vi "Modes of operation.vi"(8 "error in (no error)":errorcluster, 9 "W/R":enum16{"Write", "Read"}(ring), 10 "Ring":i8(ring) items=["No mode change/no mode assigned"=0, "Profile position mode"=1, "Velocity mode"=2, "Profile velocity mode"=3, "Torque profile mode"=4, "Homing mode"=6, "Interpolated position mode"=7, "Cyclic synchronous position mode"=8, "Cyclic synchronous velocity mode"=9, "Cyclic synchronous torque mode"=10], 11 "Motor Base in":refnum<class "Motor Base.lvclass">) -> (0 "error out":errorcluster, 2 "Ring":i8(ring) items=["No mode change/no mode assigned"=0, "Profile position mode"=1, "Velocity mode"=2, "Profile velocity mode"=3, "Torque profile mode"=4, "Homing mode"=6, "Interpolated position mode"=7, "Cyclic synchronous position mode"=8, "Cyclic synchronous velocity mode"=9, "Cyclic synchronous torque mode"=10], 3 "Motor Base out":refnum<class "Motor Base.lvclass">)   [LabVIEW 2016, in "Motor Base.lvlib" / "Motor Base.lvclass"]
uses:
  Motor Base.lvclass
  Data Type.ctl
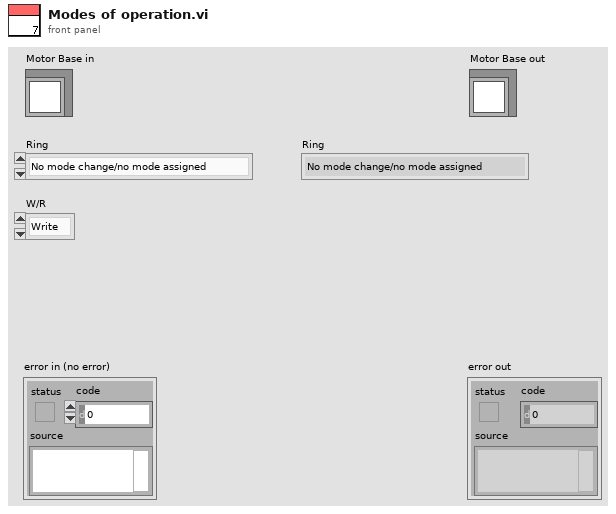
[diagram p1: front panel]
types:
  T1 = typedef "Motor Base.lvlib/Motor Base.lvclass/Data Type.ctl" = enum16{"BOOL", "I16", "I32", "I8", "OS", "U16", "U32", "U8", "VS"}
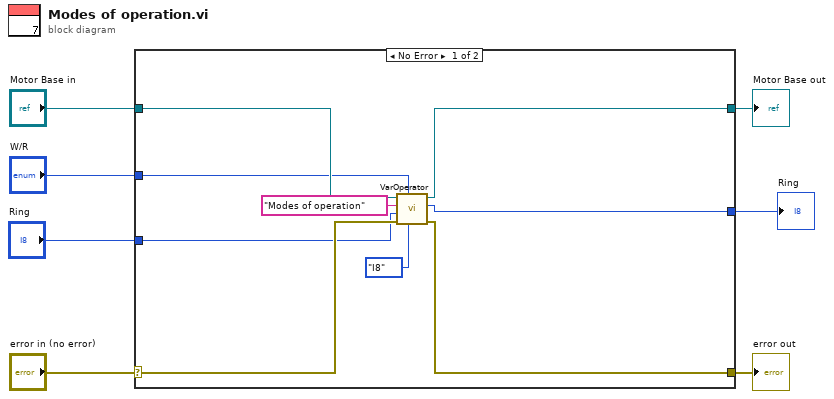
[diagram p0: block diagram]
diagram:
  n1 = case shown="No Error" "error in (no error)" {
    selector: "error in (no error)" -> [w16 w18]
    tunnel: [w15 w18] -> w6
    tunnel: [w13 w17] -> w4
    tunnel: "Motor Base in" -> [w14 w17]
    tunnel: "Ring" -> [w11 _]
    tunnel: [w10 _] -> w2
    tunnel: "W/R" -> [w8 _]
    frame No Error {
      n2 = call-dynamic "VarOperator.vi"("Data Type"=Data_Type."I8", "ro/w/r"=w8, "error in"=w16, "Data"=w11, "PDO Name"="Modes of operation", "Motor Base in"=w14) -> ("error out"=w15:errorcluster, "Data"=w10:i64, "Motor Base out"=w13:refnum<class "Motor Base.lvclass">)  [unwired: 1 in, 2 out]
    }
    frame Error {
    }
  }
  "error out" <- w6
  "Motor Base out" <- w4
  "Ring" <- w2
